vi "ALD_Main_vdP_V16.vi"() -> ()   [LabVIEW 2015]
uses:
  SubVIs and Custom Controls_V16/CTRL_Mod 7 Valve Control_V16.ctl
  SubVIs and Custom Controls_V16/CTRL_Mod 8 Valve Control_V16.ctl
  SubVIs and Custom Controls_V16/CTRL_MFC Control_V16.ctl
  SubVIs and Custom Controls_V16/CTRL_QCM Control_V16.ctl
  SubVIs and Custom Controls_V16/CTRL_Analog-In-Out-Channels_V16.ctl
  SubVIs and Custom Controls_V16/CTRL_Digital-Out-Assignments_V16.ctl
  SubVIs and Custom Controls_V16/CTRL_DO Boolean Array Cluster_V16.ctl
  SubVIs and Custom Controls_V16/CTRL_DO Arrays Precursor Process_V16.ctl
  SubVIs and Custom Controls_V16/CTRL_Analog-In Settings_V16.ctl
  <vilib>/Utility/file.llb/Read Delimited Spreadsheet (string).vi
panel:
  out "QCM Status":T1={"Crystal Status:"=FALSE, "Crystal \nLife (%)"=nan, "Mass Offset [ng/cm²]"=nan}
  in  "CLEAR GRAPHS":bool
  out "ALD Process Running?":bool
  out "Graph Start Time":timestamp=timestamp(3638646532.8725944 s since 1904-01-01) format="%<%.3X     %x>T"
  in  "Update Precursors\nReference Cluster":T2
  out "Analog-in Settings":T3={"MFC 1 Full Scale (sccm)"=200.0, "MFC 2 Full Scale (sccm)"=200.0, "MFC 3 Full Scale (sccm)"=200.0, "MFC 4 Full Scale (sccm)"=200.0, "MFC 5 Full Scale (sccm)"=200.0, "Pressure Gauge 1\nFull Scale Range (Torr)"=50.0, "Pressure Gauge 2\nFull Scale Range (Torr)"=50.0, "TC Type"=10073, "TC Units"=10143} {"TC Type" items=["J"=10072, "K"=10073, "N"=10077, "R"=10082, "S"=10085, "T"=10086, "B"=10047, "E"=10055]; "TC Units" items=["deg C"=10143, "deg F"=10144, "Kelvins"=10325, "deg R"=10145, "From Custom Scale"=10065]}
  out "error out":errorcluster
  in  "error in (no error)":errorcluster
  out "Digital Output \nAssignments":T4={"Mod 7 DAQ Name"="cDAQ1Mod7/port0", "Mod 8 DAQ Name"="cDAQ1Mod8/port0", "DO Physical Channel String"="cDAQ1Mod7/port0/line0:7, cDAQ1Mod8/port0/line0:7", "Purge DO Arrays"={"Mod7"=[FALSE, FALSE, FALSE, FALSE, FALSE, FALSE, FALSE, FALSE], "Mod8"=[FALSE, FALSE, FALSE, FALSE, FALSE, FALSE, FALSE, FALSE]}, "Hold Static DO Arrays"={"Mod7"=[TRUE, TRUE, TRUE, TRUE, TRUE, FALSE, FALSE, FALSE], "Mod8"=[TRUE, FALSE, FALSE, FALSE, FALSE, FALSE, FALSE, FALSE]}, "A1 DO Arrays"={"Pulse - Full Flow"={"Mod7"=[FALSE, FALSE, FALSE, FALSE, FALSE, FALSE, FALSE, FALSE], "Mod8"=[FALSE, TRUE, FALSE, FALSE, FALSE, FALSE, FALSE, FALSE]}, "Pulse - Diversion"={"Mod7"=[TRUE, FALSE, TRUE, TRUE, TRUE, FALSE, FALSE, FALSE], "Mod8"=[FALSE, TRUE, FALSE, FALSE, FALSE, FALSE, FALSE, FALSE]}, "Fill Chamber"={"Mod7"=[TRUE, FALSE, TRUE, TRUE, TRUE, FALSE, FALSE, FALSE], "Mod8"=[TRUE, TRUE, FALSE, FALSE, FALSE, FALSE, FALSE, FALSE]}}, "A2 DO Arrays"={"Pulse - Full Flow"={"Mod7"=[FALSE, FALSE, FALSE, FALSE, FALSE, FALSE, FALSE, FALSE], "Mod8"=[FALSE, FALSE, FALSE, FALSE, FALSE, FALSE, FALSE, FALSE]}, "Pulse - Diversion"={"Mod7"=[FALSE, FALSE, FALSE, FALSE, FALSE, FALSE, FALSE, FALSE], "Mod8"=[FALSE, FALSE, FALSE, FALSE, FALSE, FALSE, FALSE, FALSE]}, "Fill Chamber"={"Mod7"=[FALSE, FALSE, FALSE, FALSE, FALSE, FALSE, FALSE, FALSE], "Mod8"=[FALSE, FALSE, FALSE, FALSE, FALSE, FALSE, FALSE, FALSE]}}, "A3 DO Arrays"={"Pulse - Full Flow"={"Mod7"=[FALSE, FALSE, FALSE, FALSE, FALSE, FALSE, FALSE, FALSE], "Mod8"=[FALSE, FALSE, FALSE, FALSE, FALSE, FALSE, FALSE, FALSE]}, "Pulse - Diversion"={"Mod7"=[FALSE, FALSE, FALSE, FALSE, FALSE, FALSE, FALSE, FALSE], "Mod8"=[FALSE, FALSE, FALSE, FALSE, FALSE, FALSE, FALSE, FALSE]}, "Fill Chamber"={"Mod7"=[FALSE, FALSE, FALSE, FALSE, FALSE, FALSE, FALSE, FALSE], "Mod8"=[FALSE, FALSE, FALSE, FALSE, FALSE, FALSE, FALSE, FALSE]}}, "B1 DO Arrays"={"Pulse - Full Flow"={"Mod7"=[FALSE, FALSE, FALSE, FALSE, FALSE, FALSE, FALSE, FALSE], "Mod8"=[FALSE, FALSE, TRUE, FALSE, FALSE, FALSE, FALSE, FALSE]}, "Pulse - Diversion"={"Mod7"=[TRUE, TRUE, FALSE, TRUE, TRUE, FALSE, FALSE, FALSE], "Mod8"=[FALSE, FALSE, TRUE, FALSE, FALSE, FALSE, FALSE, FALSE]}, "Fill Chamber"={"Mod7"=[TRUE, TRUE, FALSE, TRUE, TRUE, FALSE, FALSE, FALSE], "Mod8"=[TRUE, FALSE, TRUE, FALSE, FALSE, FALSE, FALSE, FALSE]}}, "B2 DO Arrays"={"Pulse - Full Flow"={"Mod7"=[FALSE, FALSE, FALSE, FALSE, FALSE, FALSE, FALSE, FALSE], "Mod8"=[FALSE, FALSE, FALSE, FALSE, FALSE, FALSE, FALSE, FALSE]}, "Pulse - Diversion"={"Mod7"=[FALSE, FALSE, FALSE, FALSE, FALSE, FALSE, FALSE, FALSE], "Mod8"=[FALSE, FALSE, FALSE, FALSE, FALSE, FALSE, FALSE, FALSE]}, "Fill Chamber"={"Mod7"=[FALSE, FALSE, FALSE, FALSE, FALSE, FALSE, FALSE, FALSE], "Mod8"=[FALSE, FALSE, FALSE, FALSE, FALSE, FALSE, FALSE, FALSE]}}, "B3 DO Arrays"={"Pulse - Full Flow"={"Mod7"=[FALSE, FALSE, FALSE, FALSE, FALSE, FALSE, FALSE, FALSE], "Mod8"=[FALSE, FALSE, FALSE, FALSE, FALSE, FALSE, FALSE, FALSE]}, "Pulse - Diversion"={"Mod7"=[FALSE, FALSE, FALSE, FALSE, FALSE, FALSE, FALSE, FALSE], "Mod8"=[FALSE, FALSE, FALSE, FALSE, FALSE, FALSE, FALSE, FALSE]}, "Fill Chamber"={"Mod7"=[FALSE, FALSE, FALSE, FALSE, FALSE, FALSE, FALSE, FALSE], "Mod8"=[FALSE, FALSE, FALSE, FALSE, FALSE, FALSE, FALSE, FALSE]}}, "C1 DO Arrays"={"Pulse - Full Flow"={"Mod7"=[FALSE, FALSE, FALSE, FALSE, FALSE, FALSE, FALSE, FALSE], "Mod8"=[FALSE, FALSE, FALSE, FALSE, FALSE, FALSE, FALSE, FALSE]}, "Pulse - Diversion"={"Mod7"=[FALSE, FALSE, FALSE, FALSE, FALSE, FALSE, FALSE, FALSE], "Mod8"=[FALSE, FALSE, FALSE, FALSE, FALSE, FALSE, FALSE, FALSE]}, "Fill Chamber"={"Mod7"=[FALSE, FALSE, FALSE, FALSE, FALSE, FALSE, FALSE, FALSE], "Mod8"=[FALSE, FALSE, FALSE, FALSE, FALSE, FALSE, FALSE, FALSE]}}, "C2 DO Arrays"={"Pulse - Full Flow"={"Mod7"=[FALSE, FALSE, FALSE, FALSE, FALSE, FALSE, FALSE, FALSE], "Mod8"=[FALSE, FALSE, FALSE, TRUE, FALSE, FALSE, FALSE, FALSE]}, "Pulse - Diversion"={"Mod7"=[TRUE, TRUE, TRUE, FALSE, TRUE, FALSE, FALSE, FALSE], "Mod8"=[FALSE, FALSE, FALSE, TRUE, FALSE, FALSE, FALSE, FALSE]}, "Fill Chamber"={"Mod7"=[TRUE, TRUE, TRUE, FALSE, TRUE, FALSE, FALSE, FALSE], "Mod8"=[TRUE, FALSE, FALSE, TRUE, FALSE, FALSE, FALSE, FALSE]}}, "D1 DO Arrays"={"Pulse - Full Flow"={"Mod7"=[FALSE, FALSE, FALSE, FALSE, FALSE, FALSE, FALSE, FALSE], "Mod8"=[FALSE, FALSE, FALSE, FALSE, FALSE, FALSE, FALSE, FALSE]}, "Pulse - Diversion"={"Mod7"=[FALSE, FALSE, FALSE, FALSE, FALSE, FALSE, FALSE, FALSE], "Mod8"=[FALSE, FALSE, FALSE, FALSE, FALSE, FALSE, FALSE, FALSE]}, "Fill Chamber"={"Mod7"=[FALSE, FALSE, FALSE, FALSE, FALSE, FALSE, FALSE, FALSE], "Mod8"=[FALSE, FALSE, FALSE, FALSE, FALSE, FALSE, FALSE, FALSE]}}, "D2 DO Arrays"={"Pulse - Full Flow"={"Mod7"=[FALSE, FALSE, FALSE, FALSE, FALSE, FALSE, FALSE, FALSE], "Mod8"=[FALSE, FALSE, FALSE, FALSE, TRUE, FALSE, FALSE, FALSE]}, "Pulse - Diversion"={"Mod7"=[TRUE, TRUE, TRUE, TRUE, FALSE, FALSE, FALSE, FALSE], "Mod8"=[FALSE, FALSE, FALSE, FALSE, TRUE, FALSE, FALSE, FALSE]}, "Fill Chamber"={"Mod7"=[TRUE, TRUE, TRUE, TRUE, FALSE, FALSE, FALSE, FALSE], "Mod8"=[TRUE, FALSE, FALSE, FALSE, TRUE, FALSE, FALSE, FALSE]}}}
  out "QCM Graph":cluster{dbl[], dbl[]}[](graph)
  out "Precursor Dose Graph":cluster{dbl[], dbl[]}[](graph)
  out "Temperature Graph":cluster{dbl[], dbl[]}[](graph)
  out "MFC Graph":cluster{dbl[], dbl[]}[](graph)
  out "Pressure Graph":cluster{dbl[], dbl[]}[](graph)
  out "Process and Logging \nStatus Indicators":T7={"ALD Process Status:"="n/a", "Logging Data to:"=path "", "Process Start:"="n/a", "Process End:"="n/a", "Steps Completed:"=""}
  out "System Status Indicators":T8={"System Status:"="", "Thermocouple 1"=nan, "Thermocouple 2"=nan, "Thermocouple 3"=nan, "Thermocouple 4"=nan, "Chamber Pressure (Torr)"=nan, "Pump Pressure (Torr)"=nan} {"Pump Pressure (Torr)" scale=0.001..100.0 scale format="%.2g"; "Thermocouple 4" scale=0.0..200.0 scale format="%.1f"; "Thermocouple 3" scale=0.0..200.0 scale format="%.1f"; "Thermocouple 2" scale=0.0..200.0 scale format="%.1f"; "Chamber Pressure (Torr)" scale=0.001..100.0 scale format="%.2g"; "Thermocouple 1" scale=0.0..200.0 scale format="%.1f"}
  out "Analog In/Out \nPhysical Channels":T9={"TC 1 Name"="cDAQ1Mod1/ai0", "TC 2 Name"="cDAQ1Mod1/ai1", "TC 3 Name"="cDAQ1Mod1/ai2", "TC 4 Name"="cDAQ1Mod1/ai3", "MFC 1 Flow Name"="cDAQ1Mod2/ai0", "MFC 2 Flow Name"="cDAQ1Mod2/ai1", "MFC 3 Flow Name"="cDAQ1Mod2/ai2", "MFC 4 Flow Name"="cDAQ1Mod2/ai3", "MFC 5 Flow Name"="cDAQ1Mod2/ai4", "Pressure 1 Name"="cDAQ1Mod2/ai5", "Pressure 2 Name"="cDAQ1Mod2/ai6", "Unused AI Name"="", "MFC 1 Setpoint Name"="cDAQ1Mod4/ao0", "MFC 2 Setpoint Name"="cDAQ1Mod4/ao1", "MFC 3 Setpoint Name"="cDAQ1Mod4/ao2", "MFC 4 Setpoint Name"="cDAQ1Mod4/ao3", "MFC 5 Setpoint Name"="cDAQ1Mod5/ao0", "MKS 247 On/Off Name"="cDAQ1Mod5/ao1", "MKS 246 On/Off Name"="cDAQ1Mod5/ao2", "Unused AO Name"=""}
  out "Mod8 Indicators":T10
  out "Mod7 Indicators":T11
  in  "Run ALD process":bool
  in  "Precursors List":u16(ring) items=["None", "TMA", "H2O", "MoF6", "H2S"]
  in  "Stop Program":bool
  in  "Program Control":enum32{"Initialization", "ALD Recipe"}(tab)=enum."ALD Recipe"
  in  "MFC Control":T12 {"MFC 5 Flow" format="%.1f"; "MFC 5 setpoint" min=0.0 max=200.0 step=0.1; "MFC 4 Flow" format="%.1f"; "MFC 4 setpoint" min=0.0 max=200.0 step=0.1; "MFC 3 Flow" format="%.1f"; "MFC 3 Setpoint" min=0.0 max=200.0 step=0.1; "MFC 2 Flow" format="%.1f"; "MFC 2 Setpoint" min=0.0 max=200.0 step=0.1; "MFC 1 Flow" format="%.1f"; "MFC 1 Setpoint" min=0.0 max=200.0 step=0.1}
  in  "Module 7 \nValve Control":T13
  in  "QCM Control":T14 {"Tooling:" format="%.3g"; "Z-ratio:" format="%.3g"; "Density [g/cm²]:" format="%.3g"}
  in  "Precursors":T15={"A1"="TMA", "A2"="", "A3"="", "B1"="H2O", "B2"="", "B3"="", "C1"="", "C2"="MoF6", "D1"="", "D2"="H2S"}
  in  "Module 8 \nValve Control":T16
  in  "Data Logging":T17={"Data Log On?"=TRUE, "User:"="<Select One>", "Furnace Temp [ºC]"=nan, "Parent Directory:"=path "C:/Users/MEC104/Documents/LabView ALD Run Logs", "File Name Format:"="", "Notes:"=""} caption="(Data only logs while ALD Process is running)"
  in  "Safety Limits":T18={"Max. Chamber Press. (Torr)"=30.0, "Min. Flow (sccm)"=15.0, "Max. Flow (sccm)"=30.0, "Min. Temp (ºC)"=70.0, "Max. Temp (ºC)"=180.0, "Include MFC 1"=TRUE, "Include MFC 2"=TRUE, "Include MFC 3"=TRUE, "Include MFC 4"=TRUE, "Include MFC 5"=TRUE, "Include TC 1"=TRUE, "Include TC 2"=TRUE, "Include TC 3"=FALSE, "Include TC 4"=FALSE} {"Max. Temp (ºC)" min=0.0 step=1.0; "Min. Temp (ºC)" min=0.0 step=1.0; "Max. Flow (sccm)" min=0.0 step=1.0; "Min. Flow (sccm)" min=0.0 step=1.0; "Max. Chamber Press. (Torr)" min=0.0 step=1.0}
  in  "Process Settings":T19={"ALD Process Type:"=1, "Step 1 Precursor"=0, "Step 2 Precursor"=0, "Step 3 Precursor"=0, "Step 4 Precursor"=0, "Fill Pressure (Torr) 1"=1.5, "Fill Pressure (Torr) 2"=1.5, "Fill Pressure (Torr) 3"=1.5, "Fill Pressure (Torr) 4"=1.5, "Dose Time (s) 1"=5.0, "Dose Time (s) 2"=5.0, "Dose Time (s) 3"=5.0, "Dose Time (s) 4"=5.0, "Purge Time (s) 1"=15.0, "Purge Time (s) 2"=15.0, "Purge Time (s) 3"=15.0, "Purge Time (s) 4"=15.0, "# Loops"=10, "Add Loops"=FALSE, "# Lines"=10, "Delete lines"=FALSE, "Purge (s)"=10, "Add Purge"=FALSE, "Import table \nfrom Excel"=FALSE, "Export Table"=FALSE} {"Fill Pressure (Torr) 4" format="%.2f"; "Purge Time (s) 4" format="%.2f"; "Dose Time (s) 4" format="%.2f"; "Step 4 Precursor" items=["None", "TMA", "H2O", "MoF6", "H2S"]; "Fill Pressure (Torr) 3" format="%.2f"; "Step 3 Precursor" items=["None", "TMA", "H2O", "MoF6", "H2S"]; "Purge Time (s) 3" format="%.2f"; "Dose Time (s) 3" format="%.2f"; "Fill Pressure (Torr) 2" format="%.2f"; "Purge Time (s) 2" format="%.2f"; "Dose Time (s) 2" format="%.2f"; "Step 2 Precursor" items=["None", "TMA", "H2O", "MoF6", "H2S"]; "Fill Pressure (Torr) 1" format="%.2f"; "Dose Time (s) 1" format="%.2f"; "Purge Time (s) 1" format="%.2f"; "Step 1 Precursor" items=["None", "TMA", "H2O", "MoF6", "H2S"]; "ALD Process Type:" items=["1: Pulse-Purge (Full Flow)"=1, "2: Pulse-Purge (Diversion)"=2, "3: Fill-Hold-Purge"=3]}
  out "Execution Table":string[][](table)
  out "Execution Array":dbl[][](array[numeric])
  # "Module 7 Connections\nDigital Output (6V-30V)\n\n0:  Hold/Divert N2\n1:  Hold/Divert Manifold A\n2:  Hold/Divert Manifold B\n3:  Hold/Divert Manifold C\n4:  Hold/Divert Manifold D\n5:  Unused\n6:  Unused\n7:  Unused\n8:   V+ from 24V Power Supply\n9:   V- from 24V Power Supply"
  # "Module 8 Connections\nDigital Output (6V-30V)\n\n0:   Hold Chamber\n1:   Pulse A1\n2:   Pulse B1\n3:   Pulse C2\n4:   Pulse D2\n5:   Unused\n6:   Unused\n7:   Unused\n8:   V+ from 24V Power Supply\n9:   V- from 24V Power Supply"
  # "Analog-In:"
  # "Analog-Out:"
  # "Manifold\n(MFC #)"
  # "Setpoint\n(sccm)"
  # "Flow (sccm)"
  # "Purge (5)"
  # "D (4)"
  # "C (3)"
  # "B (2)"
  # "A (1)"
  # "Recipe \nStep"
  # "Precursor"
  # "Fill Pressure (Torr)"
  # "Dose Time \n(s)"
  # "Purge Time (s)"
  # "1"
  # "2"
  # "3"
  # "4"
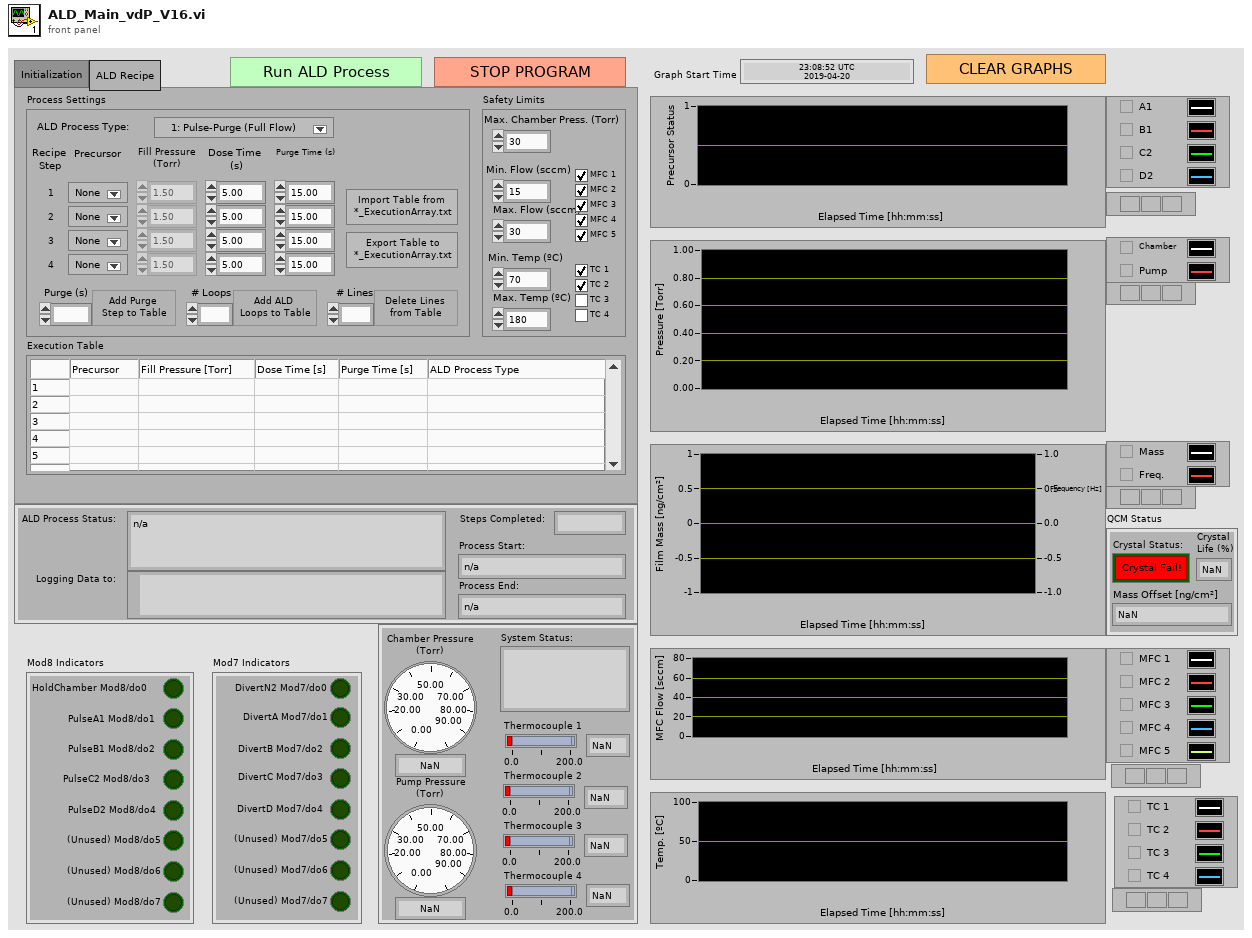
[diagram p1: front panel]
types:
  T1 = cluster{"Crystal Status:":bool, "Crystal \nLife (%)":dbl, "Mass Offset [ng/cm²]":dbl}
  T2 = cluster{"Precursors":refnum<vi>, "Precursors List":refnum<vi>, "Step 1 Precursor":refnum<vi>, "Step 2 Precursor":refnum<vi>, "Step 3 Precursor":refnum<vi>, "Step 4 Precursor":refnum<vi>, "Pulse A1":refnum<vi>, "Pulse B1":refnum<vi>, "Pulse C2":refnum<vi>, "Pulse D2":refnum<vi>}
  T3 = typedef "CTRL_Analog-In Settings_V16.ctl" = cluster{"MFC 1 Full Scale (sccm)":dbl, "MFC 2 Full Scale (sccm)":dbl, "MFC 3 Full Scale (sccm)":dbl, "MFC 4 Full Scale (sccm)":dbl, "MFC 5 Full Scale (sccm)":dbl, "Pressure Gauge 1\nFull Scale Range (Torr)":dbl, "Pressure Gauge 2\nFull Scale Range (Torr)":dbl, "TC Type":i32, "TC Units":i32}
  T4 = typedef "CTRL_Digital-Out-Assignments_V16.ctl" = cluster{"Mod 7 DAQ Name":tag, "Mod 8 DAQ Name":tag, "DO Physical Channel String":string, "Purge DO Arrays":T5, "Hold Static DO Arrays":T5, "A1 DO Arrays":T6, "A2 DO Arrays":T6, "A3 DO Arrays":T6, "B1 DO Arrays":T6, "B2 DO Arrays":T6, "B3 DO Arrays":T6, "C1 DO Arrays":T6, "C2 DO Arrays":T6, "D1 DO Arrays":T6, "D2 DO Arrays":T6}
  T5 = typedef "CTRL_DO Boolean Array Cluster_V16.ctl" = cluster{"Mod7":bool[], "Mod8":bool[]}
  T6 = typedef "CTRL_DO Arrays Precursor Process_V16.ctl" = cluster{"Pulse - Full Flow":T5, "Pulse - Diversion":T5, "Fill Chamber":T5}
  T7 = cluster{"ALD Process Status:":string, "Logging Data to:":path, "Process Start:":string, "Process End:":string, "Steps Completed:":string}
  T8 = cluster{"System Status:":string, "Thermocouple 1":dbl, "Thermocouple 2":dbl, "Thermocouple 3":dbl, "Thermocouple 4":dbl, "Chamber Pressure (Torr)":dbl, "Pump Pressure (Torr)":dbl}
  T9 = typedef "CTRL_Analog-In-Out-Channels_V16.ctl" = cluster{"TC 1 Name":tag, "TC 2 Name":tag, "TC 3 Name":tag, "TC 4 Name":tag, "MFC 1 Flow Name":tag, "MFC 2 Flow Name":tag, "MFC 3 Flow Name":tag, "MFC 4 Flow Name":tag, "MFC 5 Flow Name":tag, "Pressure 1 Name":tag, "Pressure 2 Name":tag, "Unused AI Name":tag, "MFC 1 Setpoint Name":tag, "MFC 2 Setpoint Name":tag, "MFC 3 Setpoint Name":tag, "MFC 4 Setpoint Name":tag, "MFC 5 Setpoint Name":tag, "MKS 247 On/Off Name":tag, "MKS 246 On/Off Name":tag, "Unused AO Name":tag}
  T10 = cluster{"HoldChamber Mod8/do0":bool, "PulseA1 Mod8/do1":bool, "PulseB1 Mod8/do2":bool, "PulseC2 Mod8/do3":bool, "PulseD2 Mod8/do4":bool, "(Unused) Mod8/do5":bool, "(Unused) Mod8/do6":bool, "(Unused) Mod8/do7":bool}
  T11 = cluster{"DivertN2 Mod7/do0":bool, "DivertA Mod7/do1":bool, "DivertB Mod7/do2":bool, "DivertC Mod7/do3":bool, "DivertD Mod7/do4":bool, "(Unused) Mod7/do5":bool, "(Unused) Mod7/do6":bool, "(Unused) Mod7/do7":bool}
  T12 = typedef "CTRL_MFC Control_V16.ctl" = cluster{"MFC \nFlow\nOn/Off":bool, "MFC 1 Setpoint":dbl, "MFC 2 Setpoint":dbl, "MFC 3 Setpoint":dbl, "MFC 4 setpoint":dbl, "MFC 5 setpoint":dbl, "MFC 1 Flow":dbl, "MFC 2 Flow":dbl, "MFC 3 Flow":dbl, "MFC 4 Flow":dbl, "MFC 5 Flow":dbl}
  T13 = typedef "CTRL_Mod 7 Valve Control_V16.ctl" = cluster{"Divert N2":bool, "Divert A":bool, "Divert B":bool, "Divert C":bool, "Divert D":bool}
  T14 = typedef "CTRL_QCM Control_V16.ctl" = cluster{"Film Material:":string, "Density [g/cm²]:":dbl, "Z-ratio:":dbl, "Tooling:":dbl, "QCM Monitoring":bool, "Zero Mass/Thickness":bool}
  T15 = cluster{"A1":string, "A2":string, "A3":string, "B1":string, "B2":string, "B3":string, "C1":string, "C2":string, "D1":string, "D2":string}
  T16 = typedef "CTRL_Mod 8 Valve Control_V16.ctl" = cluster{"Hold Chamber":bool, "Pulse A1":bool, "Pulse B1":bool, "Pulse C2":bool, "Pulse D2":bool}
  T17 = cluster{"Data Log On?":bool, "User:":string, "Furnace Temp [ºC]":dbl, "Parent Directory:":path, "File Name Format:":string, "Notes:":string}
  T18 = cluster{"Max. Chamber Press. (Torr)":dbl, "Min. Flow (sccm)":dbl, "Max. Flow (sccm)":dbl, "Min. Temp (ºC)":dbl, "Max. Temp (ºC)":dbl, "Include MFC 1":bool, "Include MFC 2":bool, "Include MFC 3":bool, "Include MFC 4":bool, "Include MFC 5":bool, "Include TC 1":bool, "Include TC 2":bool, "Include TC 3":bool, "Include TC 4":bool}
  T19 = cluster{"ALD Process Type:":u16, "Step 1 Precursor":u16, "Step 2 Precursor":u16, "Step 3 Precursor":u16, "Step 4 Precursor":u16, "Fill Pressure (Torr) 1":dbl, "Fill Pressure (Torr) 2":dbl, "Fill Pressure (Torr) 3":dbl, "Fill Pressure (Torr) 4":dbl, "Dose Time (s) 1":dbl, "Dose Time (s) 2":dbl, "Dose Time (s) 3":dbl, "Dose Time (s) 4":dbl, "Purge Time (s) 1":dbl, "Purge Time (s) 2":dbl, "Purge Time (s) 3":dbl, "Purge Time (s) 4":dbl, "# Loops":i32, "Add Loops":bool, "# Lines":i32, "Delete lines":bool, "Purge (s)":i32, "Add Purge":bool, "Import table \nfrom Excel":bool, "Export Table":bool}
  T20 = enum8{"Enabled", "Disabled", "Disabled and Grayed Out"}
  T21 = enum16{"open", "replace", "create", "open or create", "replace or create", "replace or create with confirmation"}
  T22 = typedef "CTRL_Digital-Out-Assignments_V15.ctl" = cluster{"Mod 7 DAQ Name":tag, "Mod 8 DAQ Name":tag, "DO Physical Channel String":string, "Purge DO Arrays":T23, "Hold Static DO Arrays":T23, "A1 DO Arrays":T24, "A2 DO Arrays":T24, "A3 DO Arrays":T24, "B1 DO Arrays":T24, "B2 DO Arrays":T24, "B3 DO Arrays":T24, "C1 DO Arrays":T24, "C2 DO Arrays":T24, "D1 DO Arrays":T24, "D2 DO Arrays":T24}
  T23 = typedef "CTRL_DO Boolean Array Cluster_V15.ctl" = cluster{"Mod7":bool[], "Mod8":bool[]}
  T24 = typedef "CTRL_DO Arrays Precursor Process_V15.ctl" = cluster{"Pulse - Full Flow":T23, "Pulse - Diversion":T23, "Fill Chamber":T23}
  T25 = cluster{"Line 1":bool, "Line 2":bool, "Line 3":bool, "Line 4":bool, "Line 0":bool}
  T26 = cluster{"ALD Process Status:":string, "Logging Data to:":path, "Process Start Time:":string, "Process End Time:":string, "Steps Completed:":string}
  T27 = cluster{"ALD Process Type:":u16, "Step 1 Precursor":u16, "Step 2 Precursor":u16, "Step 3 Precursor":u16, "Step 4 Precursor":u16, "Fill Pressure (Torr) 1":dbl, "Fill Pressure (Torr) 2":dbl, "Fill Pressure (Torr) 3":dbl, "Fill Pressure (Torr) 4":dbl, "Dose Time (s) 1":dbl, "Dose Time (s) 2":dbl, "Dose Time (s) 3":dbl, "Dose Time (s) 4":dbl, "Purge Time (s) 1":dbl, "Purge Time (s) 2":dbl, "Purge Time (s) 3":dbl, "Purge Time (s) 4":dbl, "# Loops":i32, "Add Loops":bool, "# Lines":i32, "Delete lines":bool, "Purge (s)":i32, "Add Purge":bool, "Import table \nfrom Excel":bool, "Export  table\nto Excel":bool}
  T28 = cluster{"Divert N2":bool, "Divert A":bool, "Divert B":bool, "Divert C":bool, "Divert D":bool}
  T29 = cluster{"Hold Chamber":bool, "Pulse A1":bool, "Pulse B1":bool, "Pulse C2":bool, "Pulse D2":bool}
  T30 = typedef "CTRL_Physical Channel Assignments_V14.ctl" = cluster{"TC 1 Name":tag, "TC 2 Name":tag, "TC 3 Name":tag, "TC 4 Name":tag, "MFC 1 Flow Name":tag, "MFC 2 Flow Name":tag, "MFC 3 Flow Name":tag, "MFC 4 Flow Name":tag, "MFC 5 Flow Name":tag, "Pressure 1 Name":tag, "Pressure 2 Name":tag, "Unused AI Name":tag, "MFC 1 Setpoint Name":tag, "MFC 2 Setpoint Name":tag, "MFC 3 Setpoint Name":tag, "MFC 4 Setpoint Name":tag, "MFC 5 Setpoint Name":tag, "MKS 247 On/Off Name":tag, "MKS 246 On/Off Name":tag, "Unused AO Name":tag}
  T31 = typedef "CTRL_Analog-In Settings_V14.ctl" = cluster{"MFC 1 Full Scale (sccm)":dbl, "MFC 2 Full Scale (sccm)":dbl, "MFC 3 Full Scale (sccm)":dbl, "MFC 4 Full Scale (sccm)":dbl, "MFC 5 Full Scale (sccm)":dbl, "Pressure Gauge 1\nFull Scale Range (Torr)":dbl, "Pressure Gauge 2\nFull Scale Range (Torr)":dbl, "TC Type":i32, "TC Units":i32}
  T32 = typedef "MFC Control_V13.ctl" = cluster{"MFC \nFlow\nOn/Off":bool, "MFC 1 Setpoint":dbl, "MFC 2 Setpoint":dbl, "MFC 3 Setpoint":dbl, "MFC 4 setpoint":dbl, "MFC 5 setpoint":dbl, "MFC 1 Flow":dbl, "MFC 2 Flow":dbl, "MFC 3 Flow":dbl, "MFC 4 Flow":dbl, "MFC 5 Flow":dbl}
  T33 = cluster{"Mod7 Indicators ":refnum<vi>, "Mod8 Indicators":refnum<vi>, "Module 7 \nValve Control":refnum<vi>, "Module 8 \nValve Control":refnum<vi>, "Program Control":refnum<vi>, "Execution Table":refnum<vi>, "Safety Limits":refnum<vi>, "Process Settings":refnum<vi>, "Precursors":refnum<vi>, "CLEAR GRAPHS":refnum<vi>, "Run ALD process":refnum<vi>, "ALD Process Running?":refnum<vi>, "Stop Program":refnum<vi>}
  T34 = cluster{"Graph Start Time":refnum<vi>, "Precursor Dose Graph":refnum<vi>, "Pressure Graph":refnum<vi>, "QCM Graph":refnum<vi>, "MFC Graph":refnum<vi>, "Temperature Graph":refnum<vi>}
  T35 = cluster{"Process and Logging \nStatus Indicators":refnum<vi>, "Data Logging":refnum<vi>, "MFC Control":refnum<vi>, "QCM Control":refnum<vi>, "System Status Indicators":refnum<vi>}
  T36 = cluster{"Mod7 Indicators ":refnum<vi>, "Mod8 Indicators":refnum<vi>}
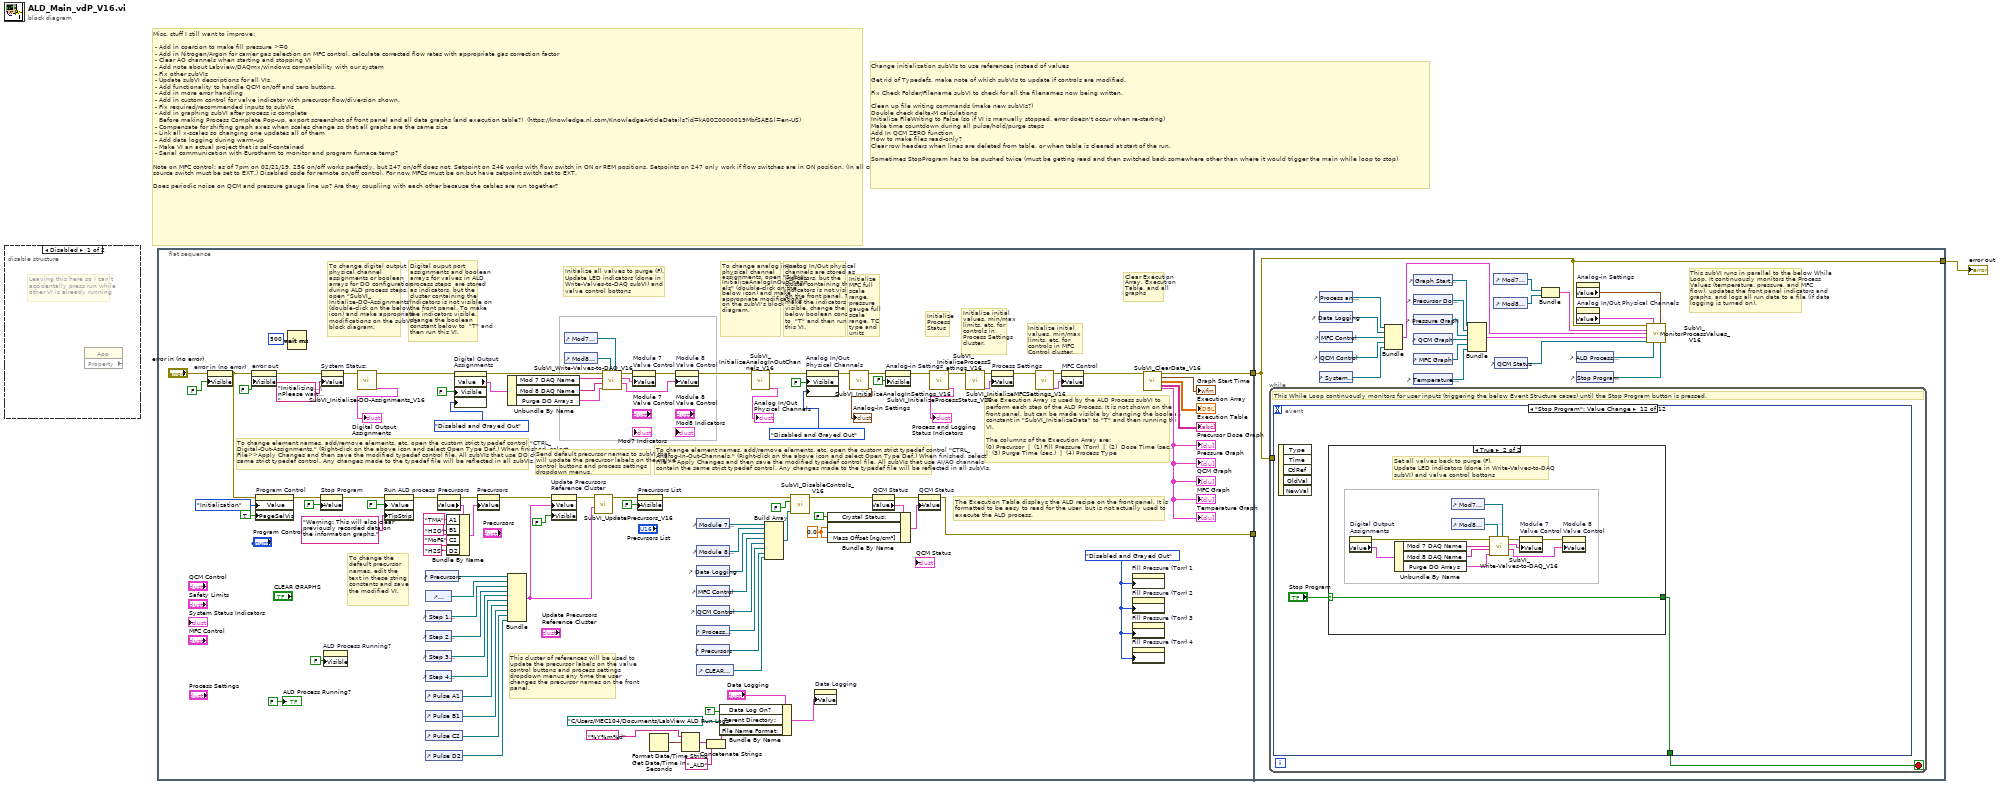
[diagram p0: block diagram]
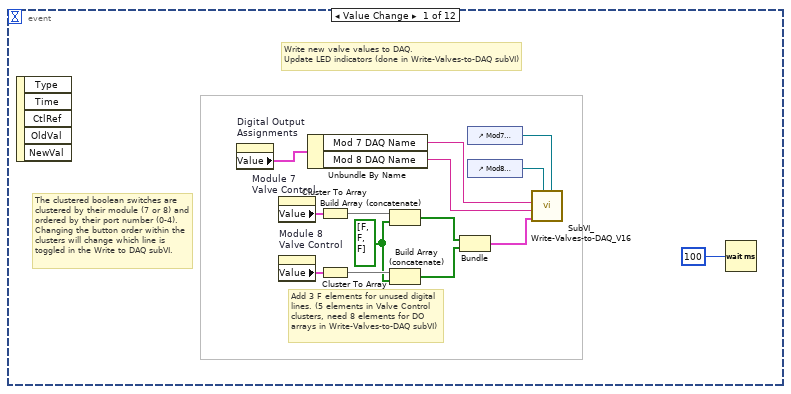
[diagram p3: hidden frame]
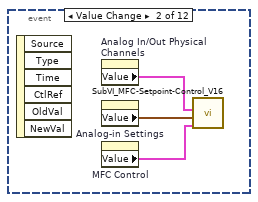
[diagram p4: hidden frame]
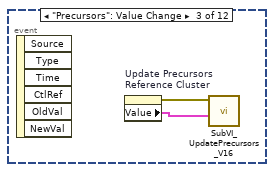
[diagram p5: hidden frame]
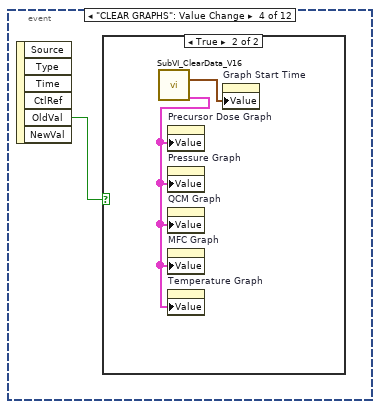
[diagram p6: hidden frame]
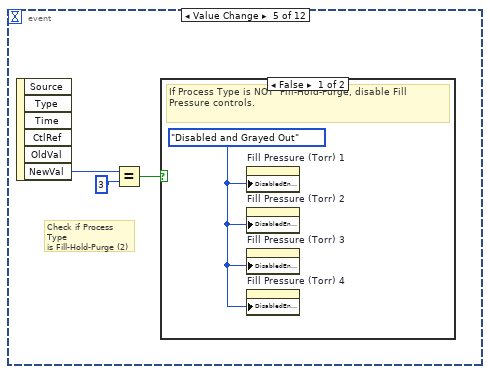
[diagram p8: hidden frame]
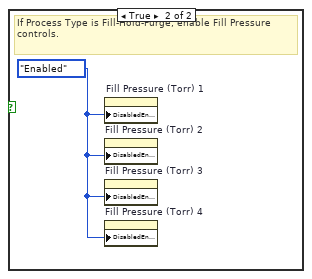
[diagram p9: hidden frame]
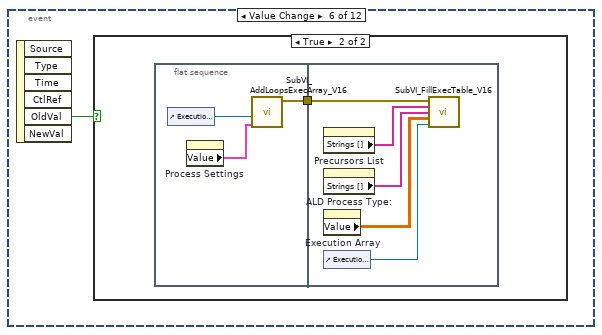
[diagram p10: hidden frame]
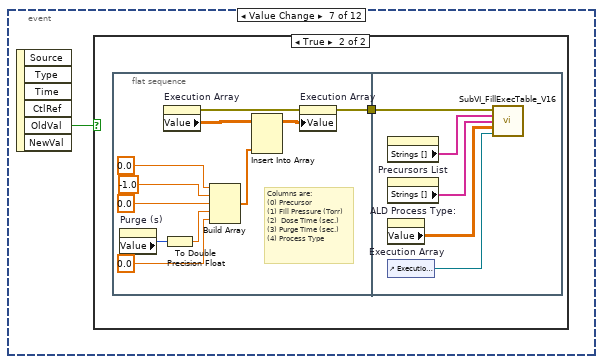
[diagram p12: hidden frame]
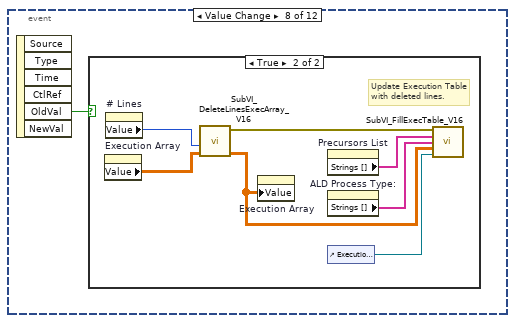
[diagram p14: hidden frame]
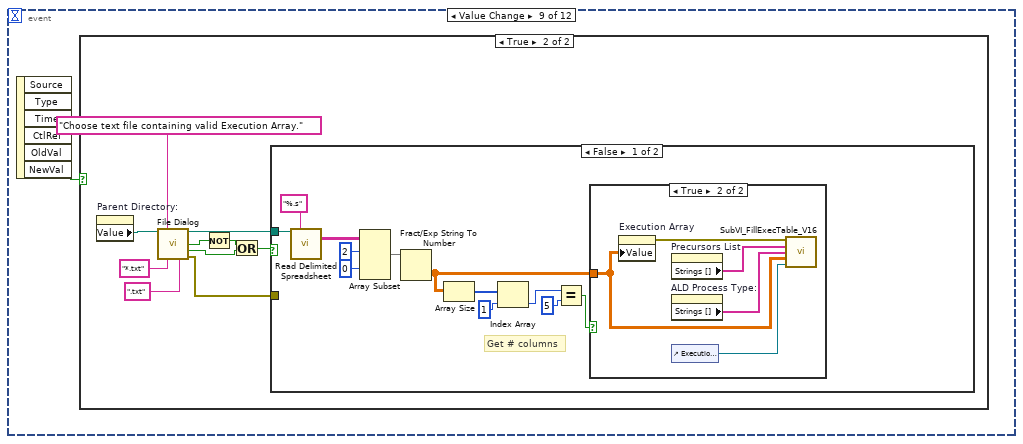
[diagram p16: hidden frame]
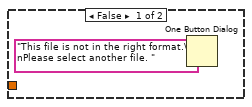
[diagram p18: hidden frame]
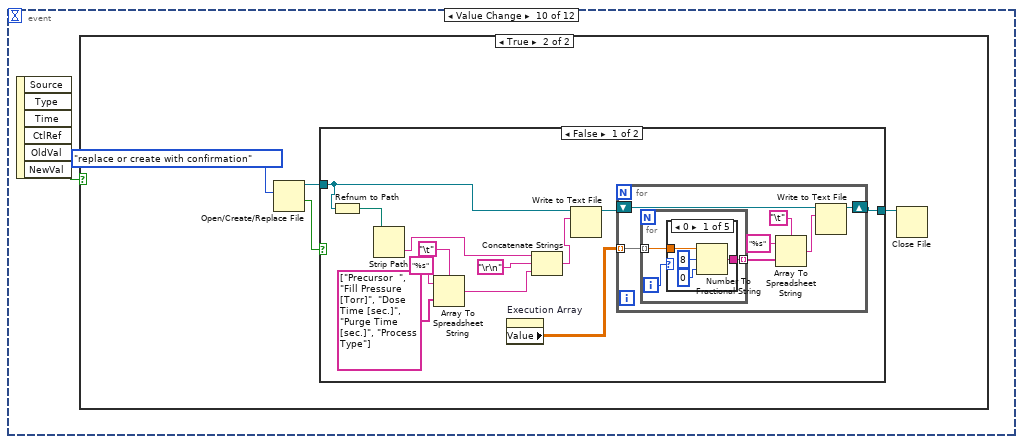
[diagram p20: hidden frame]
diagram:
  # "Change initialization subVIs to use references instead of values\n\nGet rid of Typedefs, make note of which subVIs to update if controls are modified.\n\nFix Check Folder/Filename subVI to check for all the filenames now being written.\n\nClean up file writing commands (make new subVIs?)\nDouble check delta-M calculations\nInitialize FileWriting to False (so if VI is manually stopped, error doesn't occur when re-starting)\nMake time countdown during all pulse/hold/purge steps\nAdd In QCM ZERO function\nHow to make files read-only?\nClear row headers when lines are deleted from table, or when table is cleared at start of the run.\n\nSometimes StopProgram has to be pushed twice (must be getting read and then switched back somewhere other than where it would trigger the main while loop to stop)"
  # "Misc. stuff I still want to improve:\n\n - Add in coercion to make fill pressure >=0\n - Add in Nitrogen/Argon for carrier gas selection on MFC control, calculate corrected flow rates with appropriate gas correction factor\n - Clear AO channels when starting and stopping VI\n - Add note about Labview/DAQmx/windows compatibility with our system\n - Fix other subVIs\n - Update subVI descriptions for all VIs.\n - Add functionality to handle QCM on/off and zero buttons.\n - Add in more error handling\n - Add in custom control for valve indicator with precursor flow/diversion shown.\n - Fix required/recommended inputs to subVIs\n - Add in graphing subVI after process is complete\n   Before making Process Complete Pop-up, export screenshot of front panel and all data graphs (and execution table?)  (https://knowledge.ni.com/KnowledgeArticleDetails?id=kA00Z0000019MbfSAE&l=en-US)\n - Compensate for shifting graph axes when scales change so that all graphs are the same size\n - Link all x-scales so changing one updates all of them\n - Add data logging during warm-up\n - Make VI an actual project that is self-contained\n - Serial communication with Eurotherm to monitor and program furnace temp?\n\nNote on MFC control: as of 7pm on 02/21/19, 256 on/off works perfectly, but 247 on/off does not. Setpoint on 246 works with flow switch in ON or REM positions. Setpoints on 247 only work if flow switches are in ON position. (In all cases, setpoint source switch must be set to EXT.) Disabled code for remote on/off control. For now MFCs must be on but have setpoint switch set to EXT.\n\nDoes periodic noise on QCM and pressure gauge line up? Are they coupliing with each other because the cables are run together?"
  n1 = disable-structure shown="Disabled" {
    frame Disabled {
      # "Leaving this here so I can't accidentally press run while other VI is already running"
      n2 = property class="App" props=[]() -> ()  [unwired: 2 in, 3 out]
    }
    frame Enabled {
    }
  }
  n3 = flat-sequence {
    tunnel: [w50] -> w3
    tunnel: [w23] -> w2
    tunnel: w3 -> [w111]
    tunnel: w2 -> [_]
    tunnel: [w111] -> w1
    frame #0 {
      w4 = T20."Disabled and Grayed Out" ("Disabled")
      w24 = 0.0 ("Crystal Life\nRemaining (%)")
      # "Initialize initial values, min/max limits, etc. for controls in MFC Control cluster."
      # "Send default precursor names to subVI that will update the precursor labels on the valve control buttons and process settings dropdown menus."
      # "This cluster of references will be used to update the precursor labels on the valve control buttons and process settings dropdown menus any time the user changes the precursor names on the front panel."
      # "To change the default precursor names, edit the text in these string constants and save the modified VI."
      # "Initialize Process Status"
      # "Initialize MFC full scale range, pressure gauge full scale range, TC type and units"
      # "Initialize initial values, min/max limits, etc. for controls in Process Settings cluster."
      # "The Execution Array is used by the ALD Process subVI to perform each step of the ALD Process. It is not shown on the front panel, but can be made visible by changing the boolean constant in \"SubVI_InitializeData\" to \"T\" and then running this VI.\n\nThe columns of the Execution Array are:\n(0) Precursor  |  (1) Fill Pressure (Torr)  |  (2)  Dose Time (sec.)  |  (3) Purge Time (sec.)  |  (4) Process Type"
      # "The Execution Table displays the ALD recipe on the front panel. It is formatted to be easy to read for the user, but is not actually used to execute the ALD process."
      # "Clear Execution Array, Execution Table, and all graphs"
      # "Initialize all valves to purge (F).\nUpdate LED indicators (done in Write-Valves-to-DAQ subVI) and valve control bottons"
      # "Digital ouput port assignments and boolean arrays for valves in ALD process steps  are stored as indicators, but the cluster containing the indicators is not visible on the front panel. To make the indicators visible, change the boolean constant below to  \"T\" and then run this VI."
      # "To change element names, add/remove elements, etc. open the custom strict typedef control \"CTRL_Analog-In-Out-Channels.\" (Right-click on the above icon and select Open Type Def.) When finished, select File>>Apply Changes and then save the modified typedef control file. All subVIs that use AI/AO channels contain the same strict typedef control. Any changes made to the typedef file will be reflected in all subVIs."
      # "To change element names, add/remove elements, etc. open the custom strict typedef control \"CTRL_Digital-Out-Assignments.\" (Right-click on the above icon and select Open Type Def.) When finished, select File>>Apply Changes and then save the modified typedef control file. All subVIs that use DO channels contain the same strict typedef control. Any changes made to the typedef file will be reflected in all subVIs."
      # "To change digital output physical channel assignments or boolean arrays for DO configuration during ALD process steps, open \"SubVI_Initialize-DO-Assignments\" (double-click on the below icon) and make appropriate modifications on the subVI's block diagram."
      # "To change analog in/out physical channel assignments, open \"SubVI_InitializeAnalogInOutChannels\" (double-click on the below icon) and make appropriate modifications on the subVI's block diagram."
      # "Analog In/Out physical channels are stored as indicators, but the cluster containing the indicators is not visible on the front panel. To make the indicators visible, change the below boolean constant to  \"T\" and then run this VI."
      n4 = property on="error in (no error)" class="Clust (strict)"(error in="error in (no error)", "Visible"=FALSE) -> (error out=w11:errorcluster)  [unwired: 1 in, 1 out]
      n5 = property on="error out" class="Clust (strict)"(error in=w11, "Visible"=FALSE) -> (error out=w10:errorcluster)  [unwired: 1 in, 1 out]
      n6 = property on="Program Control" class="TabCtl (strict)"(error in=w11, "Value"=enum32{"Initialization", "ALD Recipe"}."Initialization" ("Program Control"), "PageSelVis"=TRUE ("Page Selector Visible")) -> (error out=w56:errorcluster)  [unwired: 1 in, 1 out]
      n7 = Wait (ms)(milliseconds to wait=u32 500) -> ()  [unwired: 1 out]
      n8 = property on="Stop Program" class="Bool (strict)"(error in=w56, "Value"=FALSE ("stop (F)")) -> (error out=w55:errorcluster)  [unwired: 1 in, 1 out]
      n9 = property on="System Status:" class="Str"(error in=w10, "Value"="Initializing...\nPlease wait..." ("Status:")) -> (error out=w75:errorcluster)  [unwired: 1 in, 1 out]
      n10 = property on="ALD Process Running?" class="Bool (strict)"("Visible"=FALSE) -> ()  [unwired: 2 in, 2 out]
      n11 = call "SubVI_Initialize-DO-Assignments_V16.vi"("error in (no error)"=w75) -> ("Digital Output Assignments"=→"Digital Output \nAssignments":T4, "error out"=w69:errorcluster)  [unwired: 5 in]
      n12 = property on="Run ALD process" class="Bool (strict)"(error in=w55, "Value"=FALSE ("Run ALD process"), "TipStrip"="Warning: This will also clear previously recorded data on the information graphs." ("Tip Strip")) -> (error out=w54:errorcluster)  [unwired: 1 in, 1 out]
      n13 = control-ref of="Precursors"() -> (w62:refnum<vi>)
      n14 = control-ref of="Precursors List"() -> (w63:refnum<vi>)
      n15 = control-ref of="Step 1 Precursor"() -> (w76:refnum<vi>)
      n16 = control-ref of="Step 2 Precursor"() -> (w77:refnum<vi>)
      n17 = control-ref of="Step 3 Precursor"() -> (w83:refnum<vi>)
      n18 = control-ref of="Step 4 Precursor"() -> (w82:refnum<vi>)
      n19 = control-ref of="Pulse A1"() -> (w78:refnum<vi>)
      n20 = control-ref of="Pulse B1"() -> (w79:refnum<vi>)
      n21 = control-ref of="Pulse C2"() -> (w80:refnum<vi>)
      n22 = control-ref of="Pulse D2"() -> (w81:refnum<vi>)
      n23 = property on="Precursors" class="Clust (strict)"(error in=w54) -> (error out=w64:errorcluster, "Value"=w84:T15)  [unwired: 1 in, 1 out]
      n24 = Bundle By Name(cluster=w84, "A1"="TMA" ("Precursor A1"), "B1"="H2O" ("Precursor B1"), "C2"="MoF6" ("Precursor C2"), "D2"="H2S" ("Precursor D2")) -> (w65:T15)
      n25 = property on="Digital Output \nAssignments" class="Clust (strict)"(error in=w69, "Visible"=FALSE, "DisabledEnum"=T20."Disabled and Grayed Out" ("Disabled")) -> (error out=w70:errorcluster, "Value"=w68:T22)  [unwired: 1 in, 1 out]
      n26 = property on="Precursors" class="Clust (strict)"(error in=w64, "Value"=w65) -> (error out=w60:errorcluster)  [unwired: 1 in, 1 out]
      n27 = Unbundle By Name(w68) -> ("Mod 7 DAQ Name"=w30:tag, "Mod 8 DAQ Name"=w31:tag, "Purge DO Arrays"=w45:T23)
      n28 = Bundle("Precursors"=w62, "Precursors List"=w63, "Step 1 Precursor"=w76, "Step 2 Precursor"=w77, "Step 3 Precursor"=w83, "Step 4 Precursor"=w82, "Pulse A1"=w78, "Pulse B1"=w79, "Pulse C2"=w80, "Pulse D2"=w81) -> (w58:T2)  [unwired: 1 in]
      n29 = property on="Update Precursors \nReference Cluster" class="Clust (strict)"(error in=w60, "Value"=w58, "Visible"=FALSE) -> (error out=w59:errorcluster)  [unwired: 1 in, 1 out]
      n30 = control-ref of="Mod7 Indicators"() -> (w46:refnum<vi>)
      n31 = control-ref of="Mod8 Indicators"() -> (w47:refnum<vi>)
      n32 = call "SubVI_UpdatePrecursors_V16.vi"("Update Precursors\nReference Cluster"=w58, "error in (no error)"=w59) -> ("error out"=w53:errorcluster)  [unwired: 9 in]
      n33 = call "SubVI_Write-Valves-to-DAQ_V16.vi"("Mod7 Indicators Ref"=w46, "Mod8 Indicators Ref"=w47, "DO Boolean Array Cluster"=w45, "Mod8 Port Name"=w31, "Mod7 Port Name"=w30, "error in (no error)"=w70) -> ("Mod8 Buttons"=w43:T25, "Mod7 Buttons"=w99:T25, "error out"=w100:errorcluster)  [unwired: 2 in, 1 out]
      n34 = property on="Module 7 \nValve Control" class="Clust (strict)"(error in=w100, "Value"=w99) -> (error out=w44:errorcluster)  [unwired: 1 in, 1 out]
      n35 = property on="Precursors List" class="Ring (strict)"(error in=w53, "Visible"=FALSE) -> (error out=w41:errorcluster)  [unwired: 1 in, 1 out]
      n36 = Get Date/Time In Seconds() -> (seconds since 1Jan1904=w19:timestamp)
      n37 = property on="Module 8 \nValve Control" class="Clust (strict)"(error in=w44, "Value"=w43) -> (error out=w42:errorcluster)  [unwired: 1 in, 1 out]
      n38 = Format Date/Time String(time format string (%c)="%Y%m%d" ("format string"), seconds (now)=w19) -> (date/time string=w16:string)  [unwired: 1 in]
      n39 = control-ref of="Module 7 \nValve Control"() -> (w39:refnum<vi>)
      n40 = control-ref of="Module 8 \nValve Control"() -> (w38:refnum<vi>)
      n41 = control-ref of="Data Logging"() -> (w37:refnum<vi>)
      n42 = control-ref of="MFC Control"() -> (w36:refnum<vi>)
      n43 = control-ref of="QCM Control"() -> (w35:refnum<vi>)
      n44 = control-ref of="Process Settings"() -> (w34:refnum<vi>)
      n45 = control-ref of="Precursors"() -> (w33:refnum<vi>)
      n46 = control-ref of="CLEAR GRAPHS"() -> (w32:refnum<vi>)
      n47 = Concatenate Strings(w16, "_ALD") -> (w14:string)
      n48 = Bundle By Name(cluster="Data Logging", "Data Log On?"=TRUE, "Parent Directory:"=path "C:/Users/MEC104/Documents/LabView ALD Run Logs", "File Name Format:"=w14) -> (w17:T17)
      n49 = call "SubVI_InitializeAnalogInOutChannels_V16.vi"("error in (no error)"=w42) -> ("Analog In/Out Channel Assignments"=→"Analog In/Out \nPhysical Channels":T9, "error out"=w102:errorcluster)  [unwired: 5 in]
      n50 = Build Array(w39, w38, w37, w36, w35, w34, w33, w32) -> (w40:refnum<vi>[])
      n51 = call "SubVI_DisableControls_V16.vi"("appended array"=w40, "Disabled?"=FALSE, "error in (no error)"=w41) -> ("error out"=w27:errorcluster)  [unwired: 8 in]
      n52 = property on="Analog In/Out \nPhysical Channels" class="Clust (strict)"(error in=w102, "Visible"=FALSE, "DisabledEnum"=T20."Disabled and Grayed Out" ("Disabled")) -> (error out=w101:errorcluster)  [unwired: 1 in, 1 out]
      n53 = property on="Data Logging" class="Clust (strict)"("Value"=w17) -> ()  [unwired: 2 in, 2 out]
      n54 = call "SubVI_InitializeAnalogInSettings_V16.vi"("error in (no error)"=w101) -> ("Analog-in Settings"=→"Analog-in Settings":T3, "error out"=w7:errorcluster)  [unwired: 5 in]
      n55 = property on="QCM Status" class="Clust (strict)"(error in=w27) -> (error out=w26:errorcluster, "Value"=w29:T1)  [unwired: 1 in, 1 out]
      n56 = Bundle By Name(cluster=w29, "Crystal Status:"=FALSE, "Crystal \nLife (%)"=w24, "Mass Offset [ng/cm²]"=w24) -> (w28:T1)
      n57 = property on="Analog-in Settings" class="Clust (strict)"(error in=w7, "Visible"=FALSE) -> (error out=w8:errorcluster)  [unwired: 1 in, 1 out]
      n58 = property on="QCM Status" class="Clust (strict)"(error in=w26, "Value"=w28) -> (error out=w23:errorcluster)  [unwired: 1 in, 1 out]
      n59 = call "SubVI_InitializeProcessStatus_V16.vi"("error in (no error)"=w8) -> ("Process and Logging Status Indicators"=→"Process and Logging \nStatus Indicators":T26, "error out"=w52:errorcluster)  [unwired: 5 in]
      n60 = call "SubVI_InitializeProcessSettings_V16.vi"("error in (no error)"=w52) -> ("Process Settings"=w89:T27, "error out"=w90:errorcluster)  [unwired: 9 in]
      n61 = property on="Process Settings" class="Clust (strict)"(error in=w90, "Value"=w89) -> (error out=w88:errorcluster)  [unwired: 1 in, 1 out]
      n62 = call "SubVI_InitializeMFCSettings_V16.vi"("error in (no error)"=w88) -> ("MFC Control"=w86:T12, "error out"=w87:errorcluster)  [unwired: 9 in]
      n63 = property on="MFC Control" class="Clust (strict)"(error in=w87, "Value"=w86) -> (error out=w51:errorcluster)  [unwired: 1 in, 1 out]
      n64 = property on="Fill Pressure (Torr) 1" class="DigNum (strict)"("DisabledEnum"=w4) -> ()  [unwired: 2 in, 2 out]
      n65 = property on="Fill Pressure (Torr) 2" class="DigNum (strict)"("DisabledEnum"=w4) -> ()  [unwired: 2 in, 2 out]
      n66 = property on="Fill Pressure (Torr) 3" class="DigNum (strict)"("DisabledEnum"=w4) -> ()  [unwired: 2 in, 2 out]
      n67 = property on="Fill Pressure (Torr) 4" class="DigNum (strict)"("DisabledEnum"=w4) -> ()  [unwired: 2 in, 2 out]
      n68 = call "SubVI_ClearData_V16.vi"("error in (no error)"=w51) -> ("error out"=w50:errorcluster, "Time Stamp"=→"Graph Start Time":timestamp, "Empty Array"=→"Execution Array":dbl[][], "Empty Table"=→"Execution Table":string[][], "Empty Graph Data"=→"Temperature Graph" →"Precursor Dose Graph" →"Pressure Graph" →"QCM Graph" →"MFC Graph":cluster{dbl[], dbl[]}[])  [unwired: 10 in]
      "ALD Process Running?" <- FALSE ("ALD Process Running?")
    }
    frame #1 {
      # "This subVI runs in parallel to the below While Loop. It continuously monitors the Process Values (temperature, pressure, and MFC flow), updates the front panel indicators and graphs, and logs all run data to a file (if data logging is turned on)."
      n69 = while {
        tunnel: w111 -> [_]
        stop <- w133 stop-if-true
        # "This While Loop continuously monitors for user inputs (triggering the below Event Structure cases) until the Stop Program button is pressed."
        n70 = event shown="[11] \"Stop Program\": Value Change" {
          selector: _ -> [_ _ _ _ _ _ _ _ _ _ _ _]
          dyn-events: _ -> [_ _ _ _ _ _ _ _ _ _ _ _]
          timeout: _ -> [_ _ _ _ _ _ _ _ _ _ _ _]
          tunnel: [_ _ _ _ _ _ _ _ _ _ _ w320] -> w133
          event Value Change {
            w137 = bool[] [FALSE, FALSE, FALSE]
            # "Add 3 F elements for unused digital lines. (5 elements in Valve Control clusters, need 8 elements for DO arrays in Write-Valves-to-DAQ subVI)"
            # "Write new valve values to DAQ.\nUpdate LED indicators (done in Write-Valves-to-DAQ subVI)"
            # "The clustered boolean switches are clustered by their module (7 or 8) and ordered by their port number (0-4). Changing the button order within the clusters will change which line is toggled in the Write to DAQ subVI."
            n71 = event-data() -> ()  [unwired: 1 in, 5 out]
            n72 = property on="Digital Output \nAssignments" class="Clust (strict)"() -> ("Value"=w134:T22)  [unwired: 2 in, 2 out]
            n73 = property on="Module 7 \nValve Control" class="Clust (strict)"() -> ("Value"=w146:T28)  [unwired: 2 in, 2 out]
            n74 = property on="Module 8 \nValve Control" class="Clust (strict)"() -> ("Value"=w142:T29)  [unwired: 2 in, 2 out]
            n75 = Unbundle By Name(w134) -> ("Mod 7 DAQ Name"=w140:tag, "Mod 8 DAQ Name"=w143:tag)
            n76 = Cluster To Array(cluster=w146) -> (array=w139:bool[])
            n77 = Cluster To Array(cluster=w142) -> (array=w138:bool[])
            n78 = Build Array (concatenate)(w139, w137) -> (w136:bool[])
            n79 = Build Array (concatenate)(w138, w137) -> (w135:bool[])
            n80 = Bundle(w136, w135) -> (w141:cluster{bool[], bool[]})  [unwired: 1 in]
            n81 = control-ref of="Mod7 Indicators"() -> (w144:refnum<vi>)
            n82 = control-ref of="Mod8 Indicators"() -> (w145:refnum<vi>)
            n83 = call "SubVI_Write-Valves-to-DAQ_V16.vi"("Mod7 Indicators Ref"=w144, "Mod8 Indicators Ref"=w145, "DO Boolean Array Cluster"=w141, "Mod8 Port Name"=w143, "Mod7 Port Name"=w140) -> ()  [unwired: 3 in, 4 out]
            n84 = Wait (ms)(milliseconds to wait=u32 100) -> ()  [unwired: 1 out]
          }
          event Value Change {
            n85 = event-data() -> ()  [unwired: 1 in, 6 out]
            n86 = property on="Analog In/Out Physical Channels" class="Clust (strict)"() -> ("Value"=w150:T30)  [unwired: 2 in, 2 out]
            n87 = property on="Analog-in Settings" class="Clust (strict)"() -> ("Value"=w148:T31)  [unwired: 2 in, 2 out]
            n88 = property on="MFC Control" class="Clust (strict)"() -> ("Value"=w149:T32)  [unwired: 2 in, 2 out]
            n89 = call "SubVI_MFC-Setpoint-Control_V16.vi"("MFC Control"=w149, "Analog-in Settings"=w148, "Physical Channel Assignments"=w150) -> ()  [unwired: 4 in, 1 out]
          }
          event "Precursors", "Precursors.C2", "Precursors.D2", "Precursors.B1": Value Change {
            n90 = event-data() -> ()  [unwired: 1 in, 6 out]
            n91 = property on="Update Precursors\nReference Cluster" class="Clust (strict)"() -> (error out=w152:errorcluster, "Value"=w151:T2)  [unwired: 2 in, 1 out]
            n92 = call "SubVI_UpdatePrecursors_V16.vi"("Update Precursors\nReference Cluster"=w151, "error in (no error)"=w152) -> ()  [unwired: 9 in, 1 out]
          }
          event "CLEAR GRAPHS": Value Change {
            n93 = event-data() -> ("OldVal"=w153:bool)  [unwired: 1 in, 5 out]
            n94 = case shown="True" w153 {
              frame False {
              }
              frame True {
                n95 = call "SubVI_ClearData_V16.vi"() -> ("Time Stamp"=w154:timestamp, "Empty Graph Data"=w155:cluster{dbl[], dbl[]}[])  [unwired: 11 in, 3 out]
                n96 = property on="Precursor Dose Graph" class="XYGraph (strict)"("Value"=w155) -> ()  [unwired: 2 in, 2 out]
                n97 = property on="Pressure Graph" class="XYGraph (strict)"("Value"=w155) -> ()  [unwired: 2 in, 2 out]
                n98 = property on="QCM Graph" class="XYGraph (strict)"("Value"=w155) -> ()  [unwired: 2 in, 2 out]
                n99 = property on="MFC Graph" class="XYGraph (strict)"("Value"=w155) -> ()  [unwired: 2 in, 2 out]
                n100 = property on="Temperature Graph" class="XYGraph (strict)"("Value"=w155) -> ()  [unwired: 2 in, 2 out]
                n101 = property on="Graph Start Time" class="AbsTime (strict)"("Value"=w154) -> ()  [unwired: 2 in, 2 out]
              }
            }
          }
          event "Process Settings.ALD Process Type:": Value Change {
            # "Check if Process Type \nis Fill-Hold-Purge (2)"
            n102 = event-data() -> ("NewVal"=w158:u16)  [unwired: 1 in, 5 out]
            n103 = Equal?(x=w158, y=u16 3) -> (x = y?=w156:bool)
            n104 = case shown="False" w156 {
              frame False {
                w159 = T20."Disabled and Grayed Out" ("Disabled")
                # "If Process Type is NOT  Fill-Hold-Purge, disable Fill Pressure controls."
                n105 = property on="Fill Pressure (Torr) 1" class="DigNum (strict)"("DisabledEnum"=w159) -> ()  [unwired: 2 in, 2 out]
                n106 = property on="Fill Pressure (Torr) 2" class="DigNum (strict)"("DisabledEnum"=w159) -> ()  [unwired: 2 in, 2 out]
                n107 = property on="Fill Pressure (Torr) 3" class="DigNum (strict)"("DisabledEnum"=w159) -> ()  [unwired: 2 in, 2 out]
                n108 = property on="Fill Pressure (Torr) 4" class="DigNum (strict)"("DisabledEnum"=w159) -> ()  [unwired: 2 in, 2 out]
              }
              frame True {
                w160 = T20."Enabled" ("Disabled")
                # "If Process Type is Fill-Hold-Purge, enable Fill Pressure controls."
                n109 = property on="Fill Pressure (Torr) 1" class="DigNum (strict)"("DisabledEnum"=w160) -> ()  [unwired: 2 in, 2 out]
                n110 = property on="Fill Pressure (Torr) 2" class="DigNum (strict)"("DisabledEnum"=w160) -> ()  [unwired: 2 in, 2 out]
                n111 = property on="Fill Pressure (Torr) 3" class="DigNum (strict)"("DisabledEnum"=w160) -> ()  [unwired: 2 in, 2 out]
                n112 = property on="Fill Pressure (Torr) 4" class="DigNum (strict)"("DisabledEnum"=w160) -> ()  [unwired: 2 in, 2 out]
              }
            }
          }
          event "Process Settings.Add Loops": Value Change {
            n113 = event-data() -> ("OldVal"=w161:bool)  [unwired: 1 in, 5 out]
            n114 = case shown="True" w161 {
              frame False {
                # "This case is needed to handle the mechanical switching of the Add to Table button control for the Value Change event structure. \n\nWhen a boolean button is used within an event structure, the boolean control's terminal is typically placed directly within the event structure. \n\nSince the Add to Table control is contained in a cluster, its terminal does not appear explicitly on the block diagram and cannot be placed within the event structure. \n\nAdding the True/False case structure compensates for this by only executing code when the control is pressed/True, and then doing nothing when the control switches back to False."
              }
              frame True {
                n115 = flat-sequence {
                  tunnel: [w163] -> w162
                  tunnel: w162 -> [w166]
                  frame #0 {
                    n116 = control-ref of="Execution Array"() -> (w164:refnum<vi>)
                    n117 = property on="Process Settings" class="Clust (strict)"() -> ("Value"=w165:T19)  [unwired: 2 in, 2 out]
                    n118 = call "SubVI_AddLoopsExecArray_V16.vi"("Process Settings"=w165, "Execution Array"=w164) -> ("error out"=w163:errorcluster)  [unwired: 9 in]
                  }
                  frame #1 {
                    n119 = property on="Precursors List" class="Ring (strict)"() -> ("Strings []"=w168:string[])  [unwired: 2 in, 2 out]
                    n120 = property on="ALD Process Type:" class="Ring (strict)"() -> ("Strings []"=w167:string[])  [unwired: 2 in, 2 out]
                    n121 = property on="Execution Array" class="Arr (strict)"() -> ("Value"=w170:dbl[][])  [unwired: 2 in, 2 out]
                    n122 = control-ref of="Execution Table"() -> (w169:refnum<vi>)
                    n123 = call "SubVI_FillExecTable_V16.vi"("error in (no error)"=w166, "Precursors List"=w168, "Process Type"=w167, "Exec Array"=w170, "Execution Table"=w169) -> ()  [unwired: 10 in, 1 out]
                  }
                }
              }
            }
          }
          event "Process Settings.Add Purge": Value Change {
            n124 = event-data() -> ("OldVal"=w171:bool)  [unwired: 1 in, 5 out]
            n125 = case shown="True" w171 {
              frame False {
                # "This case is needed to handle the mechanical switching of the Add to Table button control for the Value Change event structure. \n\nWhen a boolean button is used within an event structure, the boolean control's terminal is typically placed directly within the event structure. \n\nSince the Add to Table control is contained in a cluster, its terminal does not appear explicitly on the block diagram and cannot be placed within the event structure. \n\nAdding the True/False case structure compensates for this by only executing code when the control is pressed/True, and then doing nothing when the control switches back to False."
              }
              frame True {
                n126 = flat-sequence {
                  tunnel: [w177] -> w172
                  tunnel: w172 -> [w184]
                  frame #0 {
                    # "Columns are:\n(0) Precursor\n(1) Fill Pressure (Torr)\n(2)  Dose Time (sec.)\n(3) Purge Time (sec.)\n(4) Process Type"
                    n127 = property on="Purge (s)" class="DigNum (strict)"() -> ("Value"=w175:i32)  [unwired: 2 in, 2 out]
                    n128 = property on="Execution Array" class="Arr (strict)"() -> (error out=w176:errorcluster, "Value"=w182:dbl[][])  [unwired: 2 in, 1 out]
                    n129 = To Double Precision Float(number=w175) -> (double precision float=w174:dbl)
                    n130 = Build Array(0.0 ("element"), -1.0 ("element"), 0.0 ("element"), w174, 0.0 ("element")) -> (w183:dbl[])
                    n131 = Insert Into Array(array=w182, new element=w183) -> (w173:dbl[][])  [unwired: 2 in]
                    n132 = property on="Execution Array" class="Arr (strict)"(error in=w176, "Value"=w173) -> (error out=w177:errorcluster)  [unwired: 1 in, 1 out]
                  }
                  frame #1 {
                    n133 = property on="Precursors List" class="Ring (strict)"() -> ("Strings []"=w186:string[])  [unwired: 2 in, 2 out]
                    n134 = property on="ALD Process Type:" class="Ring (strict)"() -> ("Strings []"=w185:string[])  [unwired: 2 in, 2 out]
                    n135 = property on="Execution Array" class="Arr (strict)"() -> ("Value"=w188:dbl[][])  [unwired: 2 in, 2 out]
                    n136 = control-ref of="Execution Table"() -> (w187:refnum<vi>)
                    n137 = call "SubVI_FillExecTable_V16.vi"("error in (no error)"=w184, "Precursors List"=w186, "Process Type"=w185, "Exec Array"=w188, "Execution Table"=w187) -> ()  [unwired: 10 in, 1 out]
                  }
                }
              }
            }
          }
          event "Process Settings.Delete lines": Value Change {
            n138 = event-data() -> ("OldVal"=w189:bool)  [unwired: 1 in, 5 out]
            n139 = case shown="True" w189 {
              frame False {
                # "This case is needed to handle the mechanical switching of the Delete Lines button control for the Value Change event structure. \n\nWhen a boolean button is used within an event structure, the boolean control's terminal is typically placed directly within the event structure. \n\nSince the Delete Lines control is contained in a cluster, its terminal does not appear explicitly on the block diagram and cannot be placed within the event structure. \n\nAdding the True/False case structure compensates for this by only executing code when the control is pressed/True, and then doing nothing when the control switches back to False."
              }
              frame True {
                # "Update Execution Table with deleted lines."
                n140 = property on="Execution Array" class="Arr (strict)"() -> ("Value"=w193:dbl[][])  [unwired: 2 in, 2 out]
                n141 = property on="# Lines" class="DigNum (strict)"() -> ("Value"=w192:i32)  [unwired: 2 in, 2 out]
                n142 = call "SubVI_DeleteLinesExecArray_V16.vi"("Input Array"=w193, "# Lines to Delete"=w192) -> ("Output Array"=w191:dbl[][], "error out"=w190:errorcluster)  [unwired: 8 in]
                n143 = property on="Execution Array" class="Arr (strict)"("Value"=w191) -> ()  [unwired: 2 in, 2 out]
                n144 = property on="Precursors List" class="Ring (strict)"() -> ("Strings []"=w195:string[])  [unwired: 2 in, 2 out]
                n145 = property on="ALD Process Type:" class="Ring (strict)"() -> ("Strings []"=w194:string[])  [unwired: 2 in, 2 out]
                n146 = control-ref of="Execution Table"() -> (w196:refnum<vi>)
                n147 = call "SubVI_FillExecTable_V16.vi"("error in (no error)"=w190, "Precursors List"=w195, "Process Type"=w194, "Exec Array"=w191, "Execution Table"=w196) -> ()  [unwired: 10 in, 1 out]
              }
            }
          }
          event "Process Settings.Import table \nfrom Excel": Value Change {
            n148 = event-data() -> ("OldVal"=w197:bool)  [unwired: 1 in, 5 out]
            n149 = case shown="True" w197 {
              frame False {
                # "This case is needed to handle the mechanical switching of the Import Table from Excel button control for the Value Change event structure. \n\nWhen a boolean button is used within an event structure, the boolean control's terminal is typically placed directly within the event structure. \n\nSince the Import Table from Excel control is contained in a cluster, its terminal does not appear explicitly on the block diagram and cannot be placed within the event structure. \n\nAdding the True/False case structure compensates for this by only executing code when the control is pressed/True, and then doing nothing when the control  automatically switches back to False."
              }
              frame True {
                n150 = property on="Parent Directory:" class="Path"() -> ("Value"=w205:path)  [unwired: 2 in, 2 out]
                n151 = call "File Dialog"("start path"=w205, "prompt"="Choose text file containing valid Execution Array.", "pattern (all files)"="*.txt", "pattern label"=".txt") -> ("selected path"=w207:path, "exists"=w202:bool, "cancelled"=w200:bool, "error out"=w206:errorcluster)  [unwired: 8 in]
                n152 = Not(x=w202) -> (.not. x?=w201:bool)
                n153 = Or(x=w201, y=w200) -> (x .or. y?=w199:bool)
                n154 = case shown="False" w199 {
                  tunnel: w207 -> [w216 _]
                  tunnel: w206 -> [_ _]
                  frame False {
                    # "Get # columns"
                    n155 = call-poly <vilib>:"Read Delimited Spreadsheet.vi"("file path (dialog if empty)"=w216, "format (%s)"="%.s" ("format (%.3f)")) -> ("all rows"=w214:string[][])  [unwired: 8 in, 5 out]
                    n156 = Array Subset(array=w214, index (row)=2 ("index"), index (col)=0 ("index")) -> (w211:string[][])  [unwired: 2 in]
                    n157 = Fract/Exp String To Number(string=w211) -> (number=w208:dbl[][])  [unwired: 3 in, 1 out]
                    n158 = Array Size(array=w208) -> (size(s)=w210:i32[])
                    n159 = Index Array(array=w210, index=1) -> (element=w209:i32)
                    n160 = Equal?(x=w209, y=5) -> (x = y?=w218:bool)
                    n161 = case shown="True" w218 {
                      tunnel: w208 -> [_ w223]
                      frame False {
                        n162 = One Button Dialog(message="This file is not in the right format.\nPlease select another file. ") -> ()  [unwired: 1 in, 1 out]
                      }
                      frame True {
                        n163 = property on="Execution Array" class="Arr (strict)"("Value"=w223) -> (error out=w221:errorcluster)  [unwired: 2 in, 1 out]
                        n164 = property on="Precursors List" class="Ring (strict)"() -> ("Strings []"=w224:string[])  [unwired: 2 in, 2 out]
                        n165 = property on="ALD Process Type:" class="Ring (strict)"() -> ("Strings []"=w222:string[])  [unwired: 2 in, 2 out]
                        n166 = control-ref of="Execution Table"() -> (w225:refnum<vi>)
                        n167 = call "SubVI_FillExecTable_V16.vi"("error in (no error)"=w221, "Precursors List"=w224, "Process Type"=w222, "Exec Array"=w223, "Execution Table"=w225) -> ()  [unwired: 10 in, 1 out]
                      }
                    }
                  }
                  frame True {
                  }
                }
              }
            }
          }
          event "Process Settings.Export Table": Value Change {
            n168 = event-data() -> ("OldVal"=w226:bool)  [unwired: 1 in, 5 out]
            n169 = case shown="True" w226 {
              frame False {
                # "This case is needed to handle the mechanical switching of the Import Table from Excel button control for the Value Change event structure. \n\nWhen a boolean button is used within an event structure, the boolean control's terminal is typically placed directly within the event structure. \n\nSince the Import Table from Excel control is contained in a cluster, its terminal does not appear explicitly on the block diagram and cannot be placed within the event structure. \n\nAdding the True/False case structure compensates for this by only executing code when the control is pressed/True, and then doing nothing when the control  automatically switches back to False."
              }
              frame True {
                n170 = Open/Create/Replace File(operation (0:open)=T21."replace or create with confirmation") -> (refnum out=w230:refnum<file>, cancelled=w227:bool)  [unwired: 5 in, 1 out]
                n171 = case shown="False" w227 {
                  tunnel: w230 -> [w232 w273]
                  tunnel: [w236 w273] -> w229
                  frame False {
                    n172 = Refnum to Path(1:w232) -> (0:w231:path)
                    n173 = Strip Path(path=w231) -> (name=w234:string)  [unwired: 1 out]
                    n174 = Array To Spreadsheet String(delimiter (Tab)="\t", array=string[] ["Precursor  ", "Fill Pressure [Torr]", "Dose Time [sec.]", "Purge Time [sec.]", "Process Type"], 3:"%s" ("format string")) -> (spreadsheet string=w242:string)
                    n175 = property on="Execution Array" class="Arr (strict)"() -> ("Value"=w235:dbl[][])  [unwired: 2 in, 2 out]
                    n176 = Concatenate Strings(w234, "\r\n", w242) -> (w239:string)
                    n177 = Write to Text File(file (use dialog)=w232, text=w239) -> (refnum out=w237:refnum<file>)  [unwired: 2 in, 2 out]
                    n178 = for {
                      tunnel: w235 -> [w243] mode=indexing
                      shift-right: [w244] -> w236
                      shift-left: w237 -> [w247]
                      n179 = for {
                        tunnel: [w251] -> w249 mode=indexing
                        tunnel: w243 -> [w250] mode=indexing
                        i -> [w252]
                        n180 = case shown="0" w252 {
                          tunnel: w250 -> [w256 w260 w264 w268 w272]
                          tunnel: [w253 w257 w261 w265 w269] -> w251
                          frame 0 {
                            n181 = Number To Fractional String(number=w256, width (-)=i16 8, precision (6)=i16 0) -> (F-format string=w253:string)  [unwired: 1 in]
                          }
                          frame 1, Default {
                            n182 = Number To Fractional String(number=w260, width (-)=i16 8, precision (6)=i16 2) -> (F-format string=w257:string)  [unwired: 1 in]
                          }
                          frame 2 {
                            n183 = Number To Fractional String(number=w264, width (-)=i16 8, precision (6)=i16 2) -> (F-format string=w261:string)  [unwired: 1 in]
                          }
                          frame 3 {
                            n184 = Number To Fractional String(number=w268, width (-)=i16 8, precision (6)=i16 2) -> (F-format string=w265:string)  [unwired: 1 in]
                          }
                          frame 4 {
                            n185 = Number To Fractional String(number=w272, width (-)=i16 8, precision (6)=i16 0) -> (F-format string=w269:string)  [unwired: 1 in]
                          }
                        }
                      }
                      n186 = Array To Spreadsheet String(delimiter (Tab)="\t", array=w249, 3:"%s" ("format string")) -> (spreadsheet string=w245:string)
                      n187 = Write to Text File(file (use dialog)=w247, text=w245) -> (refnum out=w244:refnum<file>)  [unwired: 2 in, 2 out]
                    }
                  }
                  frame True {
                  }
                }
                n188 = Close File(refnum=w229) -> ()  [unwired: 1 in, 2 out]
              }
            }
          }
          event "Run ALD process": Value Change {
            n189 = event-data() -> ()  [unwired: 1 in, 5 out]
            n190 = property on="Execution Array" class="Arr (strict)"() -> ("Value"=w274:dbl[][])  [unwired: 2 in, 2 out]
            n191 = property on="Data Log On?" class="Bool (strict)"() -> ("Value"=w275:bool)  [unwired: 2 in, 2 out]
            n192 = case shown="True" "Run ALD process" {
              tunnel: w275 -> [_ w281]
              tunnel: w274 -> [_ w278]
              frame False {
              }
              frame True {
                n193 = case shown="True" w281 {
                  tunnel: [TRUE w285] -> w280
                  frame False {
                  }
                  frame True {
                    n194 = control-ref of="Data Logging"() -> (w284:refnum<vi>)
                    n195 = control-ref of="Run ALD process"() -> (w283:refnum<vi>)
                    n196 = call "SubVI_CheckFolderFileName_V16.vi"("Run ALD process Ref"=w283, "Data Logging"=w284) -> ("Folder and \nFile Name OK?"=w285:bool)  [unwired: 8 in, 1 out]
                  }
                }
                n197 = call "SubVI_CheckExecArray_V16.vi"("Exec Array"=w278) -> ("Array OK"=w277:bool)  [unwired: 9 in, 1 out]
                n198 = And(x=w280, y=w277) -> (x .and. y?=w279:bool)
                n199 = case shown="True" w279 {
                  tunnel: w277 -> [w286 _]
                  frame False {
                    n200 = case shown="False" w286 {
                      frame False {
                        # "If the Execution Array is empty or contains invalid values, alert the user but do not start the ALD Process."
                        n201 = flat-sequence {
                          frame #0 {
                            n202 = property on="Run ALD process" class="Bool (strict)"("Value"=FALSE ("Run ALD process")) -> ()  [unwired: 2 in, 2 out]
                          }
                          frame #1 {
                            n203 = One Button Dialog(message="Invalid Execution Table.\nUse the ALD Recipe Setup tab to populate the Execution Table, then press Run. ") -> ()  [unwired: 1 in, 1 out]
                          }
                        }
                      }
                      frame True {
                        # "If Execution Array is OK, then Invalid file/folder options were chose. CheckFolderAndFile subVI prevents process execution, so no action is needed here."
                      }
                    }
                  }
                  frame True {
                    # "If the Execution Array is not empty and no problems exist with Data Logging settings, start the ALD Process."
                    n204 = control-ref of="Mod7 Indicators"() -> (w304:refnum<vi>)
                    n205 = control-ref of="Mod8 Indicators"() -> (w303:refnum<vi>)
                    n206 = control-ref of="Module 7 \nValve Control"() -> (w302:refnum<vi>)
                    n207 = control-ref of="Module 8 \nValve Control"() -> (w301:refnum<vi>)
                    n208 = control-ref of="Program Control"() -> (w300:refnum<vi>)
                    n209 = control-ref of="Execution Table"() -> (w299:refnum<vi>)
                    n210 = control-ref of="Safety Limits"() -> (w298:refnum<vi>)
                    n211 = control-ref of="Process Settings"() -> (w297:refnum<vi>)
                    n212 = control-ref of="Precursors"() -> (w296:refnum<vi>)
                    n213 = control-ref of="CLEAR GRAPHS"() -> (w295:refnum<vi>)
                    n214 = control-ref of="Run ALD process"() -> (w294:refnum<vi>)
                    n215 = control-ref of="ALD Process Running?"() -> (w293:refnum<vi>)
                    n216 = control-ref of="Stop Program"() -> (w292:refnum<vi>)
                    n217 = Bundle("Mod7 Indicators"=w304, "Mod8 Indicators"=w303, "Module 7 \nValve Control"=w302, "Module 8 \nValve Control"=w301, "Program Control"=w300, "Execution Table"=w299, "Safety Limits"=w298, "Process Settings"=w297, "Precursors"=w296, "CLEAR GRAPHS"=w295, "Run ALD process"=w294, "ALD Process Running?"=w293, "Stop Program"=w292) -> (w291:T33)  [unwired: 1 in]
                    n218 = control-ref of="Process and Logging \nStatus Indicators"() -> (w314:refnum<vi>)
                    n219 = control-ref of="Data Logging"() -> (w312:refnum<vi>)
                    n220 = control-ref of="MFC Control"() -> (w313:refnum<vi>)
                    n221 = control-ref of="QCM Control"() -> (w311:refnum<vi>)
                    n222 = control-ref of="System Status Indicators"() -> (w315:refnum<vi>)
                    n223 = control-ref of="Graph Start Time"() -> (w305:refnum<vi>)
                    n224 = control-ref of="Precursor Dose Graph"() -> (w306:refnum<vi>)
                    n225 = control-ref of="Pressure Graph"() -> (w307:refnum<vi>)
                    n226 = control-ref of="QCM Graph"() -> (w308:refnum<vi>)
                    n227 = control-ref of="MFC Graph"() -> (w309:refnum<vi>)
                    n228 = control-ref of="Temperature Graph"() -> (w310:refnum<vi>)
                    n229 = Bundle("Graph Start Time"=w305, "Precursor Dose Graph"=w306, "Pressure Graph"=w307, "QCM Graph"=w308, "MFC Graph"=w309, "Temperature Graph"=w310) -> (w289:T34)  [unwired: 1 in]
                    n230 = Bundle("Process and Logging \nStatus Indicators"=w314, "Data Logging"=w312, "MFC Control"=w313, "QCM Control"=w311, "System Status Indicators"=w315) -> (w290:T35)  [unwired: 1 in]
                    n231 = property on="Digital Output \nAssignments" class="Clust (strict)"() -> ("Value"=w318:T22)  [unwired: 2 in, 2 out]
                    n232 = property on="Execution Array" class="Arr (strict)"() -> ("Value"=w317:dbl[][])  [unwired: 2 in, 2 out]
                    n233 = property on="Precursors List" class="Ring (strict)"() -> ("Strings []"=w316:string[])  [unwired: 2 in, 2 out]
                    n234 = call "SubVI_ALD-Process_V16.vi"("Precursors List (Strings)"=w316, "Digital Output Assignments"=w318, "output cluster"=w290, "output cluster 4"=w291, "Graph Ref Cluster"=w289, "Exec Array"=w317) -> ()  [unwired: 9 in, 1 out]
                  }
                }
              }
            }
          }
          event "Stop Program": Value Change {
            n235 = event-data() -> ()  [unwired: 1 in, 5 out]
            n236 = case shown="True" "Stop Program" {
              selector: "Stop Program" -> [w321 w333]
              tunnel: [w321 w333] -> w320
              frame False {
              }
              frame True {
                # "Set all valves back to purge (F).\nUpdate LED indicators (done in Write-Valves-to-DAQ subVI) and valve control bottons"
                n237 = property on="Digital Output \nAssignments" class="Clust (strict)"() -> (error out=w326:errorcluster, "Value"=w325:T22)  [unwired: 2 in, 1 out]
                n238 = Unbundle By Name(w325) -> ("Mod 7 DAQ Name"=w324:tag, "Mod 8 DAQ Name"=w323:tag, "Purge DO Arrays"=w322:T23)
                n239 = control-ref of="Mod7 Indicators"() -> (w329:refnum<vi>)
                n240 = control-ref of="Mod8 Indicators"() -> (w330:refnum<vi>)
                n241 = call "SubVI_Write-Valves-to-DAQ_V16.vi"("Mod7 Indicators Ref"=w329, "Mod8 Indicators Ref"=w330, "DO Boolean Array Cluster"=w322, "Mod8 Port Name"=w323, "Mod7 Port Name"=w324, "error in (no error)"=w326) -> ("Mod8 Buttons"=w327:T25, "Mod7 Buttons"=w331:T25, "error out"=w332:errorcluster)  [unwired: 2 in, 1 out]
                n242 = property on="Module 7 \nValve Control" class="Clust (strict)"(error in=w332, "Value"=w331) -> (error out=w328:errorcluster)  [unwired: 1 in, 1 out]
                n243 = property on="Module 8 \nValve Control" class="Clust (strict)"(error in=w328, "Value"=w327) -> ()  [unwired: 1 in, 2 out]
              }
            }
          }
        }
      }
      n244 = control-ref of="Process and Logging \nStatus Indicators"() -> (w122:refnum<vi>)
      n245 = control-ref of="Data Logging"() -> (w114:refnum<vi>)
      n246 = control-ref of="MFC Control"() -> (w115:refnum<vi>)
      n247 = control-ref of="QCM Control"() -> (w113:refnum<vi>)
      n248 = control-ref of="System Status Indicators"() -> (w128:refnum<vi>)
      n249 = Bundle("Process and Logging \nStatus Indicators"=w122, "Data Logging"=w114, "MFC Control"=w115, "QCM Control"=w113, "System Status Indicators"=w128) -> (w116:T35)  [unwired: 1 in]
      n250 = control-ref of="Graph Start Time"() -> (w120:refnum<vi>)
      n251 = control-ref of="Precursor Dose Graph"() -> (w123:refnum<vi>)
      n252 = control-ref of="Pressure Graph"() -> (w124:refnum<vi>)
      n253 = control-ref of="QCM Graph"() -> (w125:refnum<vi>)
      n254 = control-ref of="MFC Graph"() -> (w126:refnum<vi>)
      n255 = control-ref of="Temperature Graph"() -> (w127:refnum<vi>)
      n256 = Bundle("Graph Start Time"=w120, "Precursor Dose Graph"=w123, "Pressure Graph"=w124, "QCM Graph"=w125, "MFC Graph"=w126, "Temperature Graph"=w127) -> (w130:T34)  [unwired: 1 in]
      n257 = control-ref of="Mod7 Indicators"() -> (w119:refnum<vi>)
      n258 = control-ref of="Mod8 Indicators"() -> (w118:refnum<vi>)
      n259 = control-ref of="QCM Status"() -> (w112:refnum<vi>)
      n260 = Bundle("Mod7 Indicators"=w119, "Mod8 Indicators"=w118) -> (w117:T36)  [unwired: 1 in]
      n261 = property on="Analog-in Settings" class="Clust (strict)"() -> ("Value"=w121:T31)  [unwired: 2 in, 2 out]
      n262 = property on="Analog In/Out Physical Channels" class="Clust (strict)"() -> ("Value"=w129:T30)  [unwired: 2 in, 2 out]
      n263 = control-ref of="ALD Process Running?"() -> (w131:refnum<vi>)
      n264 = control-ref of="Stop Program"() -> (w132:refnum<vi>)
      n265 = call "SubVI_MonitorProcessValues_V16.vi"("error in"=w111, "Physical Channel Assignments"=w129, "Analog-in Settings"=w121, "Valve Indicators"=w117, "Front Panel Controls and Indicators Refnum Cluster"=w116, "Front Panel Graph RefCluster"=w130, "QCM Status"=w112, "ALD Process Running?"=w131, "Stop Program Refnum"=w132) -> ()  [unwired: 6 in, 1 out]
    }
  }
  "error out" <- w1
